vi "Turbine Flow.vi"(0 "Structure Width (m)":u32, 2 "Energy Needed (FE)":u32, 5 "Rotor Height (m)":u32, 11 "Stored Gas (mB/t)":u32, 12 "Blades":u32, 13 "Coils":u32, 14 "Vents":u32) -> (4 "Flow (mB/t)":u32, 6 "Vents Limiting":bool, 8 "Dispersers Limiting":bool, 10 "Blades Limiting":bool, 15 "Coils Limiting":bool)   [LabVIEW 2021]
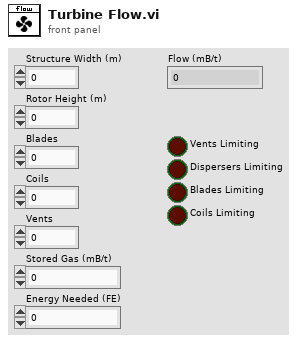
[diagram p1: front panel]
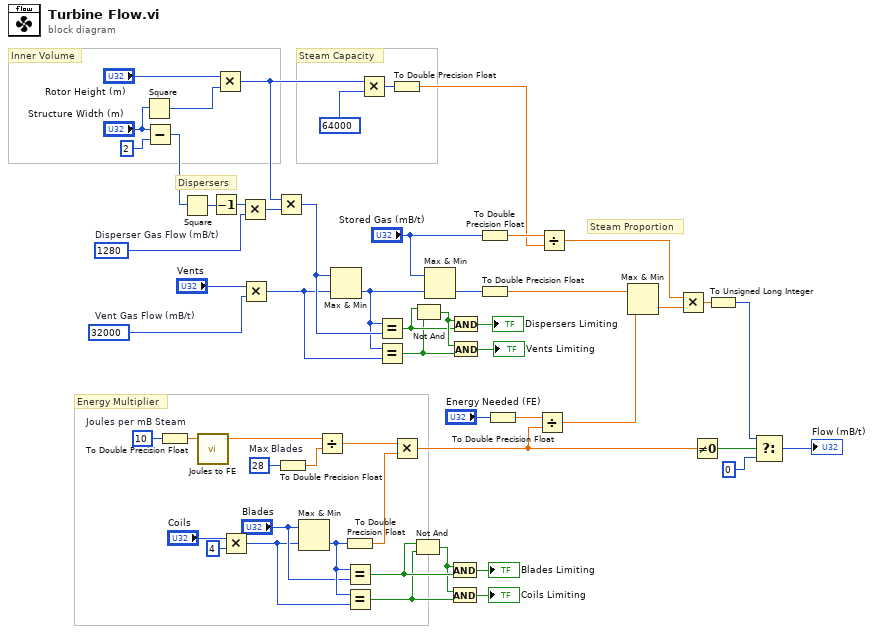
[diagram p0: block diagram]
diagram:
  w48 = u32 28  # Max Blades
  w50 = u32 10  # Joules per mB Steam
  w52 = u32 32000  # Vent Gas Flow (mB/t)
  w54 = u32 1280  # Disperser Gas Flow (mB/t)
  # "Dispersers"
  # "Steam Proportion"
  # "Steam Capacity"
  # "Energy Multiplier"
  # "Inner Volume"
  n1 = Square(x="Structure Width (m)") -> (x^2=w15:u32)
  n2 = Subtract(x="Structure Width (m)", y=u32 2) -> (x-y=w24:u32)
  n3 = To Double Precision Float(number=w50) -> (double precision float=w2:dbl)
  n4 = Square(x=w24) -> (x^2=w26:u32)
  n5 = call "Joules to FE.vi"("J"=w2) -> ("FE"=w1:ext)  [unwired: 4 in]
  n6 = Decrement(x=w26) -> (x-1=w25:u32)
  n7 = Multiply(x="Rotor Height (m)", y=w15) -> (x*y=w3:u32)
  n8 = Multiply(x="Coils", y=u32 4) -> (x*y=w16:u32)
  n9 = Multiply(x=w25, y=w54) -> (x*y=w51:u32)
  n10 = Multiply(x="Vents", y=w52) -> (x*y=w19:u32)
  n11 = Multiply(x=w3, y=w51) -> (x*y=w21:u32)
  n12 = To Double Precision Float(number=w48) -> (double precision float=w49:dbl)
  n13 = Max & Min(x="Blades", y=w16) -> (min(x,y)=w18:u32)  [unwired: 1 out]
  n14 = Divide(x=w1, y=w49) -> (x/y=w47:ext)
  n15 = Max & Min(x=w21, y=w19) -> (min(x,y)=w20:u32)  [unwired: 1 out]
  n16 = To Double Precision Float(number=w18) -> (double precision float=w44:dbl)
  n17 = Equal?(x=w18, y="Blades") -> (x = y?=w14:bool)
  n18 = Equal?(x=w18, y=w16) -> (x = y?=w11:bool)
  n19 = Multiply(x=w3, y=u32 64000) -> (x*y=w34:u32)
  n20 = Equal?(x=w20, y=w21) -> (x = y?=w8:bool)
  n21 = Equal?(x=w20, y=w19) -> (x = y?=w7:bool)
  n22 = To Double Precision Float(number=w34) -> (double precision float=w33:dbl)
  n23 = Multiply(x=w47, y=w44) -> (x*y=w37:ext)
  n24 = Not And(1:w11, 2:w14) -> (0:w12:bool)
  n25 = Not And(1:w7, 2:w8) -> (0:w9:bool)
  n26 = Max & Min(x="Stored Gas (mB/t)", y=w20) -> (min(x,y)=w40:u32)  [unwired: 1 out]
  n27 = And(x=w12, y=w14) -> (x .and. y?=→"Blades Limiting":bool)
  n28 = And(x=w12, y=w11) -> (x .and. y?=→"Coils Limiting":bool)
  n29 = And(x=w9, y=w8) -> (x .and. y?=→"Dispersers Limiting":bool)
  n30 = And(x=w9, y=w7) -> (x .and. y?=→"Vents Limiting":bool)
  n31 = To Double Precision Float(number="Stored Gas (mB/t)") -> (double precision float=w35:dbl)
  n32 = To Double Precision Float(number=w40) -> (double precision float=w32:dbl)
  n33 = To Double Precision Float(number="Energy Needed (FE)") -> (double precision float=w38:dbl)
  n34 = Divide(x=w38, y=w37) -> (x/y=w29:ext)
  n35 = Divide(x=w35, y=w33) -> (x/y=w31:dbl)
  n36 = Max & Min(x=w32, y=w29) -> (min(x,y)=w30:ext)  [unwired: 1 out]
  n37 = Multiply(x=w31, y=w30) -> (x*y=w22:ext)
  n38 = Not Equal To 0?(x=w37) -> (x != 0?=w43:bool)
  n39 = To Unsigned Long Integer(number=w22) -> (unsigned 32bit integer=w27:u32)
  n40 = Select(t=w27, s=w43, f=u32 0 ("Stored Gas (mB/t)")) -> (s? t:f=→"Flow (mB/t)":u32)
